vi "Error Handler Queue.vi"(11 "Error Handler Queue":refnum<class "Message Enqueuer.lvclass">) -> (3 "Error Handler Queue Out":refnum<class "Message Enqueuer.lvclass">)   [LabVIEW 2015, in "Mag Lab Error Handler.lvlib" / "Mag Lab Error Handler.lvclass"]
uses:
  Mag Lab Error Handler.lvclass
  <vilib>/ActorFramework/Message Enqueuer/Message Enqueuer.lvclass
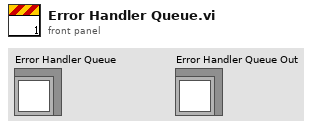
[diagram p1: front panel]
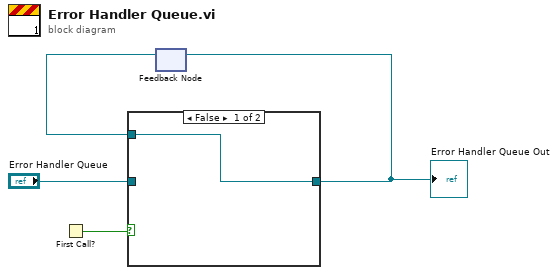
[diagram p0: block diagram]
diagram:
  n1 = First Call?() -> (First Call?: T/F=w4:bool)
  n2 = feedback #1() -> (w1:refnum<class "Message Enqueuer.lvclass">)  [unwired: 1 in]
  n3 = case shown="False" w4 {
    tunnel: "Error Handler Queue" -> [_ w6]
    tunnel: [w5 w6] -> w2
    tunnel: w1 -> [w5 _]
    frame False {
    }
    frame True {
    }
  }
  "Error Handler Queue Out" <- w2
  n4 = feedback-in #1(w2) -> ()
